vi "create png.vi"(8 "error in":errorcluster, 10 "IMG_FORMAT":enum32{".png", ".jpg", ".bmp"}(ring), 11 "base path":path) -> (0 "error out":errorcluster, 3 "path":path)   [LabVIEW 2018]
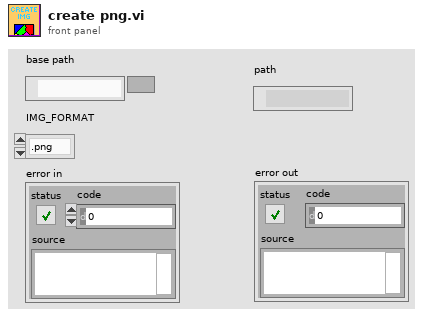
[diagram p1: front panel]
types:
  T1 = enum16{"open", "replace", "create", "open or create", "replace or create", "replace or create with confirmation"}
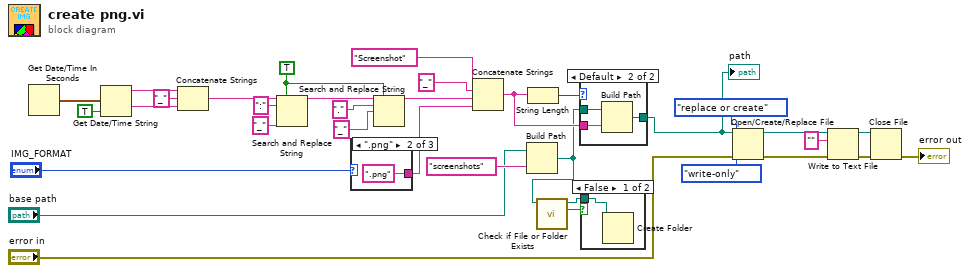
[diagram p0: block diagram]
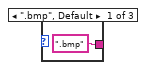
[diagram p4: hidden frame]
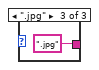
[diagram p5: hidden frame]
diagram:
  w20 = TRUE
  n1 = Get Date/Time In Seconds() -> (seconds since 1Jan1904=w12:timestamp)
  n2 = Get Date/Time String(seconds (now)=w12, want seconds? (F)=TRUE) -> (date string=w13:string, time string=w21:string)  [unwired: 1 in]
  n3 = Concatenate Strings(w13, "_" ("string"), w21) -> (w14:string)
  n4 = Search and Replace String(replace all?=w20, input string=w14, search string=":", replace string="_" ("replace string (\"\")")) -> (result string=w17:string)  [unwired: 4 in, 3 out]
  n5 = case shown="\".png\"" "IMG_FORMAT" {
    tunnel: [".bmp" ("name or relative path") ".png" ("name or relative path") ".jpg" ("name or relative path")] -> w24
    frame ".bmp", Default {
    }
    frame ".png" {
    }
    frame ".jpg" {
    }
  }
  n6 = Search and Replace String(replace all?=w20, input string=w17, search string=".", replace string="_" ("replace string (\"\")")) -> (result string=w9:string)  [unwired: 4 in, 3 out]
  n7 = Concatenate Strings("Screenshot" ("name or relative path"), "_" ("name or relative path"), w9, w24) -> (w26:string)
  n8 = Build Path(base path="base path", name or relative path="screenshots") -> (appended path=w3:path)
  n9 = String Length(string=w26) -> (length=w25:i32)
  n10 = call <vilib>:"Check if File or Folder Exists.vi"("path"=w3) -> ("file or folder exists?"=w2:bool, "dup path"=w1:path)  [unwired: 8 in, 1 out]
  n11 = case shown="Default" w25 {
    tunnel: [w38 w41] -> w7
    tunnel: w3 -> [w38 w40]
    tunnel: w26 -> [_ w39]
    frame 0 {
    }
    frame Default {
      n12 = Build Path(base path=w40, name or relative path=w39) -> (appended path=w41:path)
    }
  }
  "path" <- w7
  n13 = case shown="False" w2 {
    tunnel: w1 -> [w42 _]
    frame False {
      n14 = Create Folder(path (use dialog)=w42) -> ()  [unwired: 2 in, 3 out]
    }
    frame True {
    }
  }
  n15 = Open/Create/Replace File(file path (use dialog)=w7, error in="error in", operation (0:open)=T1."replace or create", access (0:read/write)=enum16{"read/write", "read-only", "write-only"}."write-only") -> (refnum out=w32:refnum<file>, error out=w33:errorcluster)  [unwired: 2 in, 1 out]
  n16 = Write to Text File(file (use dialog)=w32, text="", error in=w33) -> (refnum out=w31:refnum<file>, error out=w30:errorcluster)  [unwired: 1 in, 1 out]
  n17 = Close File(refnum=w31, error in=w30) -> (error out=→"error out":errorcluster)  [unwired: 1 out]
